vi "Synchronize TDC.vi"(8 "error in":errorcluster, 11 "References In":T1[](array[typedef])) -> (0 "error out":errorcluster, 2 "Current TE Phase":i32[](array[numeric]), 3 "References Out":T1[](array[typedef]))   [LabVIEW 2011, in "FlexRIO Host Library (User).lvlib"]
uses:
  FlexRIO Host Library (User).lvlib
  <vilib>/rvi/interface/nirviReadWriteControl/nirviReadWriteControl.xnode
  Session/FPGA Session Ref.ctl
  Zeiss Acquisition Demo/FPGA Bitfiles/FlexRIODigitizer_FPGABoard_Acquire_Rev2.lvbitx
  <vilib>/rvi/errors/niLvFpgaMergeErrorWithErrorCode.vi
  <vilib>/rvi/errors/niLvFpgaAdjustHostInterfaceError.vi
panel:
  in  "trigger enable period":fxp<+,9,9>=50.0
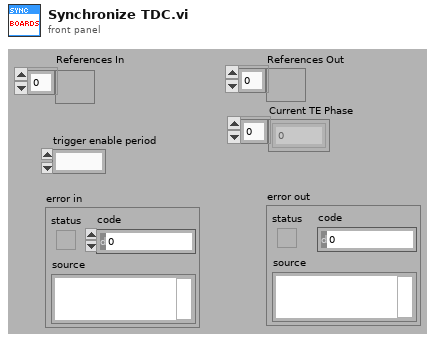
[diagram p1: front panel]
types:
  T1 = typedef "FlexRIO Host.lvlib/FPGA Session Ref.ctl" = refnum<k20>
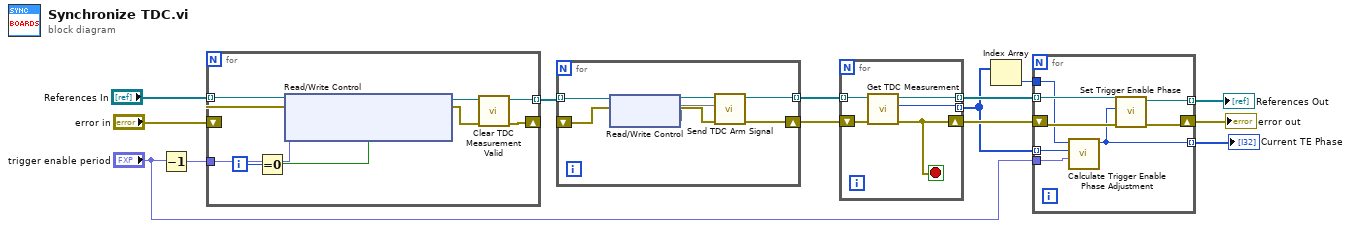
[diagram p0: block diagram]
diagram:
  n1 = Decrement(x="trigger enable period") -> (x-1=w4:fxp<+,9,9>)
  n2 = for {
    tunnel: "References In" -> [w23] mode=indexing
    shift-right: [w16] -> _
    shift-left: "error in" -> [w22]
    tunnel: w4 -> [w21]
    tunnel: [w15] -> w1 mode=indexing
    i -> [w20]
    n3 = Equal To 0?(x=w20) -> (x = 0?=w19:bool)
    n4 = xnode "Read/Write Control"("FPGA VI Reference In"=w23, "error in"=w22, "trigger enable period (less 1)"=w21, "is master?"=w19) -> ("FPGA VI Reference Out"=w18:T1, "error out"=w17:errorcluster)
    n5 = call "Clear TDC Measurement Valid.vi"("error in"=w17, "FPGA VI Reference In"=w18) -> ("error out"=w16:errorcluster, "FPGA VI Reference Out"=w15:T1)  [unwired: 6 in, 2 out]
  }
  n6 = for {
    tunnel: [w30] -> w12 mode=indexing
    tunnel: w1 -> [w28] mode=indexing
    shift-right: [w29] -> w14
    shift-left: _ -> [w27]
    n7 = xnode "Read/Write Control"("FPGA VI Reference In"=w28, "error in"=w27) -> ("FPGA VI Reference Out"=w26:T1, "error out"=w25:errorcluster, "is master?"=w24)
    n8 = call "Send TDC Arm Signal.vi"("error in"=w25, "master?"=w24, "FPGA VI Reference In"=w26) -> ("error out"=w29:errorcluster, "FPGA VI Reference Out"=w30:T1)  [unwired: 7 in]
  }
  n9 = for {
    tunnel: [w34] -> w11 mode=indexing
    tunnel: w12 -> [w33] mode=indexing
    shift-right: [w32] -> w13
    shift-left: w14 -> [w35]
    tunnel: [w31] -> w7 mode=indexing
    stop <- w32 stop-if-true
    n10 = call "Get TDC Measurement.vi"("error in"=w35, "FPGA VI Reference In"=w33) -> ("error out"=w32:errorcluster, "tdc measurement"=w31:u16, "FPGA VI Reference Out"=w34:T1)  [unwired: 4 in, 3 out]
  }
  n11 = Index Array(array=w7) -> (element=w8:u16)  [unwired: 1 in]
  n12 = for {
    shift-right: [w41] -> w10
    shift-left: w13 -> [w42]
    tunnel: w11 -> [w43] mode=indexing
    tunnel: [w40] -> w9 mode=indexing
    tunnel: w8 -> [w39]
    tunnel: w7 -> [w38] mode=indexing
    tunnel: "trigger enable period" -> [w37]
    tunnel: [w36] -> w2 mode=indexing
    n13 = call "Calculate Trigger Enable Phase Adjustment.vi"("trigger enable period"=w37, "slave measurement"=w38, "master measurement"=w39) -> ("trigger enable adjust amount"=w36:i32)  [unwired: 8 in]
    n14 = call "Set Trigger Enable Phase.vi"("error in"=w42, "phase value"=w36, "FPGA VI Reference In"=w43) -> ("error out"=w41:errorcluster, "FPGA VI Reference Out"=w40:T1)  [unwired: 7 in]
  }
  "References Out" <- w9
  "error out" <- w10
  "Current TE Phase" <- w2
